vi "L5K Reader Action v2.vi"(8 "error in":errorcluster, 11 "L5K File Path":path) -> (0 "error out":errorcluster, 1 "Import Error":string, 3 "L5K Information":T1)   [LabVIEW 2011]
uses:
  L5K Internal Data.ctl
  L5K Tag.ctl
  L5K Data Types.ctl
  ST Enum.ctl
  Ethernet IP Custom Device Custom Device.lvlib
panel:
  out "concatenated string":string
  in  "Import Error - String":string="\n%s - Reason: this tag is a multidimensional array. VeriStand EtherNet/IP add-on only support 1D array tags."
  in  "Import Error - Array":string="\n%s - Reason: this tag is a multidimensional array. VeriStand EtherNet/IP add-on only support 1D array tags."
  in  "Import Error - Data Type":string="\n%s - Reason: the data type of this tag is not supported by the VeriStand EtherNet/IP add-on. Enter this tag manually with a generic datatype."
  in  "Import Error":string="VeriStand EtherNet/IP add-on did not import the following tags:\n"
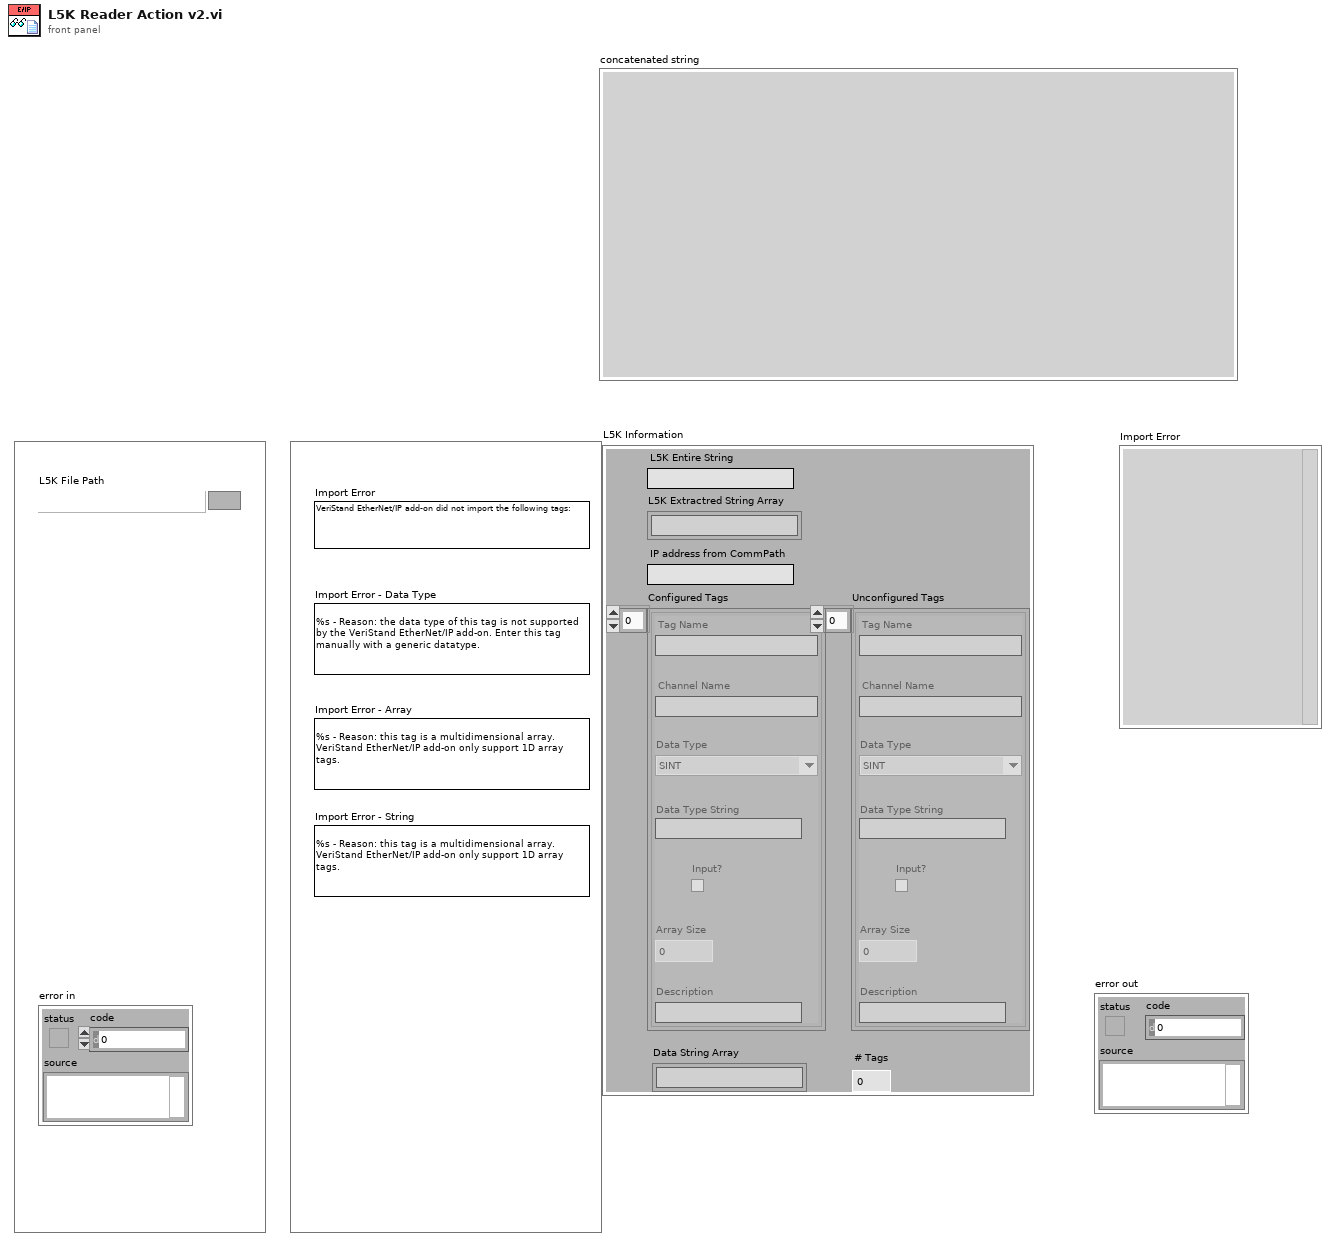
[diagram p1: front panel]
types:
  T1 = typedef "Ethernet IP Custom Device Custom Device.lvlib/L5K Internal Data.ctl" = cluster{"L5K Entire String":string, "L5K Extractred String Array":string[], "IP address from CommPath":string, "Configured Tags":T2[], "Data String Array":string[], "Unconfigured Tags":T2[], "# Tags":i32}
  T2 = typedef "Ethernet IP Custom Device Custom Device.lvlib/L5K Tag.ctl" = cluster{"Tag Name":string, "Data Type":T3, "Data Type String":string, "Array Size":i32, "Description":string, "Input?":bool, "Channel Name":string}
  T3 = typedef "Ethernet IP Custom Device Custom Device.lvlib/L5K Data Types.ctl" = enum16{"SINT", "INT", "DINT", "REAL", "BOOL"}
  T4 = typedef "Ethernet IP Custom Device Custom Device.lvlib/ST Enum.ctl" = enum16{"Init", "Extract Strings", "Extract Tags", "Exit"}
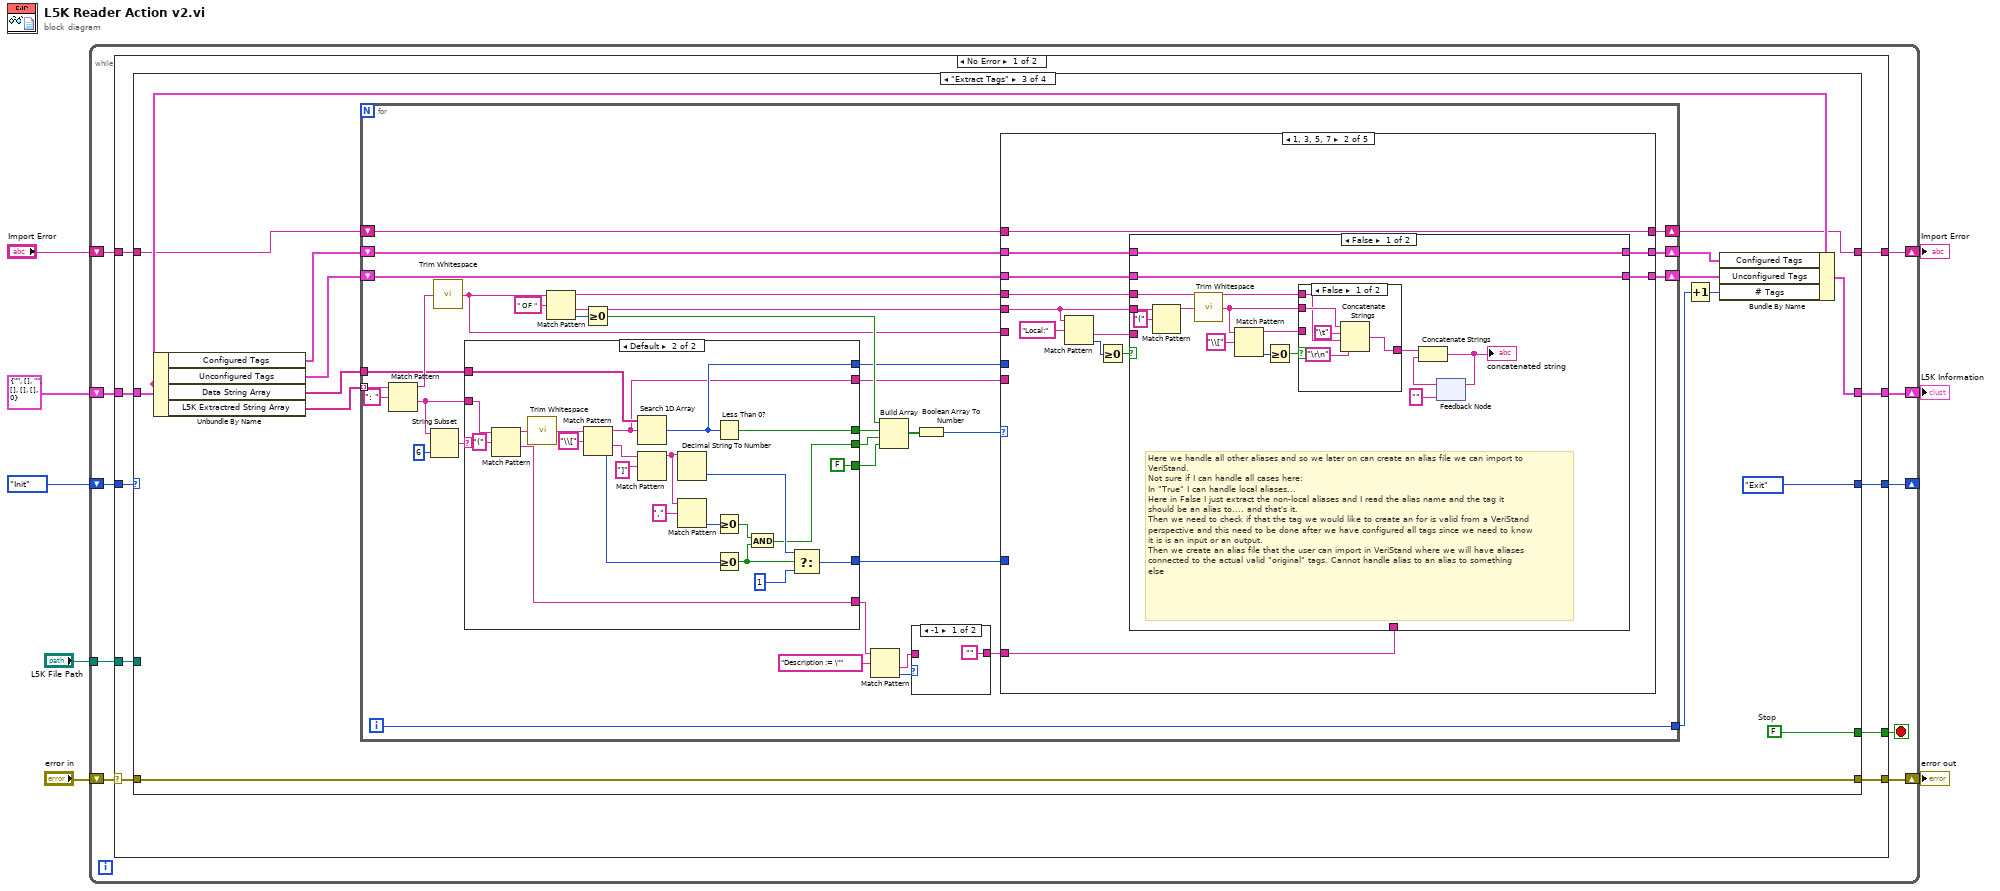
[diagram p0: block diagram]
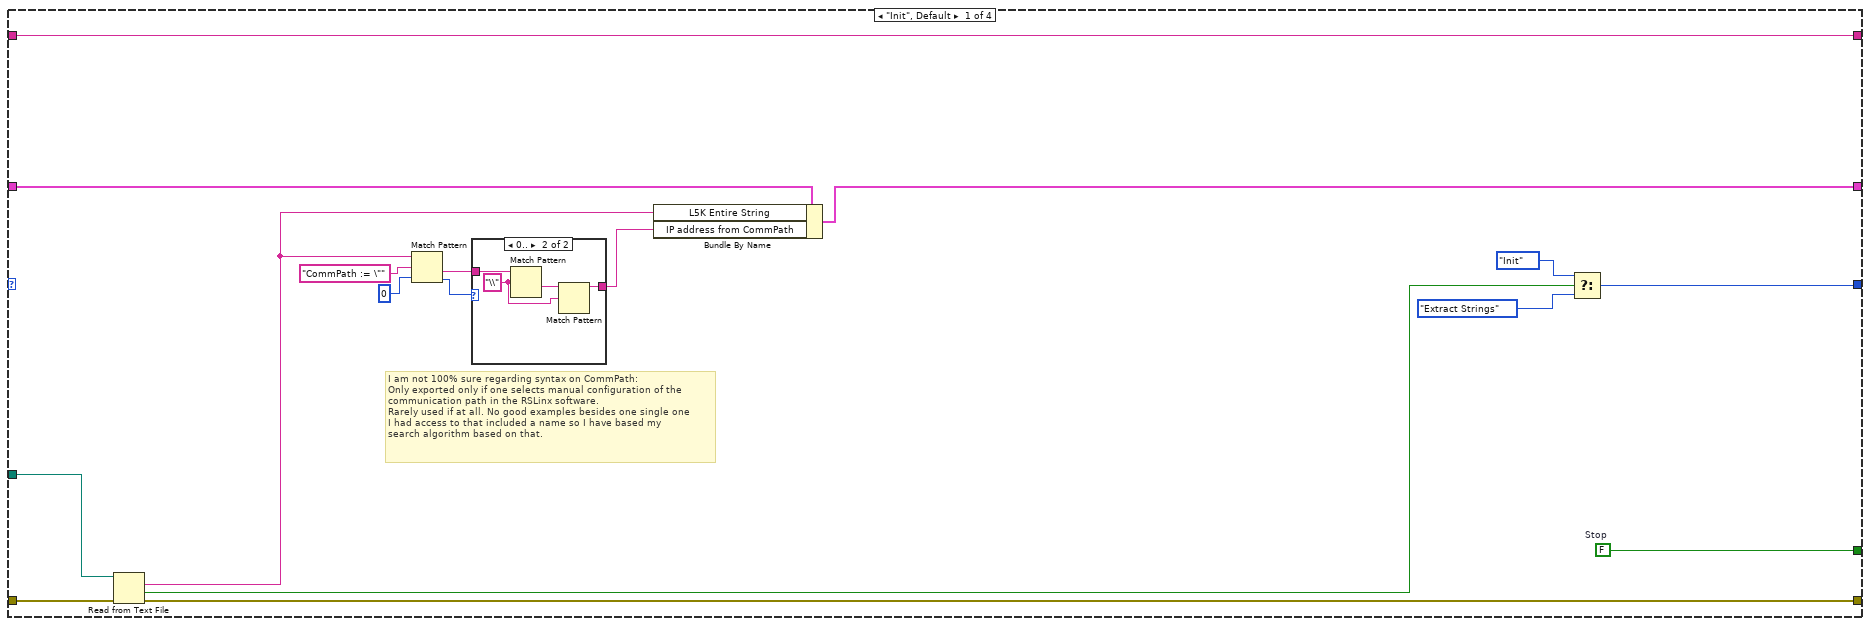
[diagram p2: hidden frame]
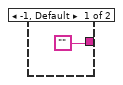
[diagram p3: hidden frame]
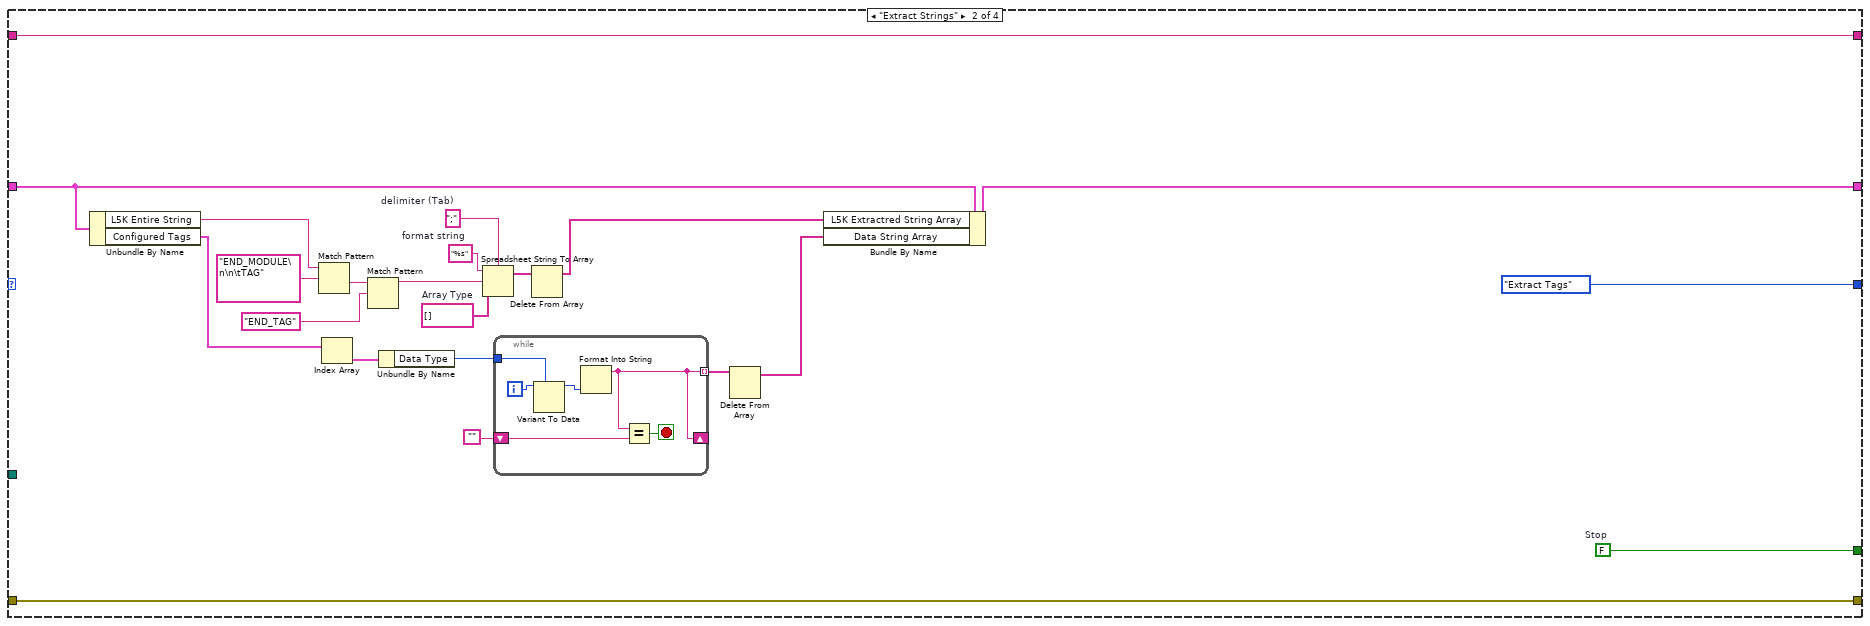
[diagram p4: hidden frame]
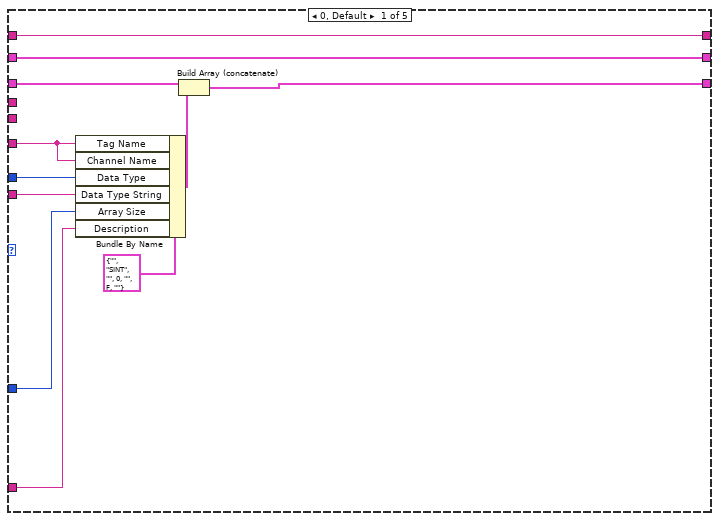
[diagram p5: hidden frame]
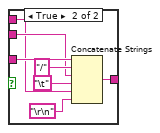
[diagram p6: hidden frame]
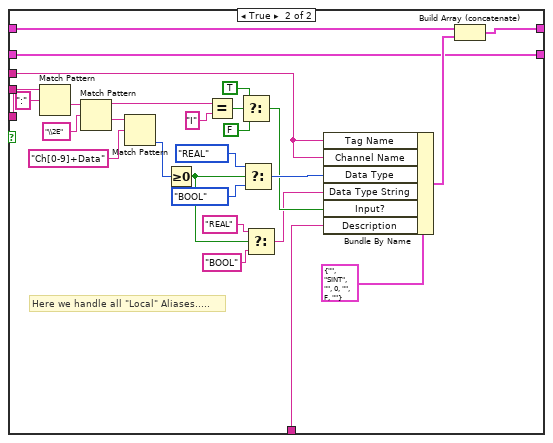
[diagram p7: hidden frame]
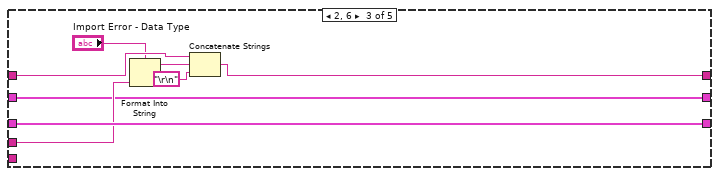
[diagram p8: hidden frame]
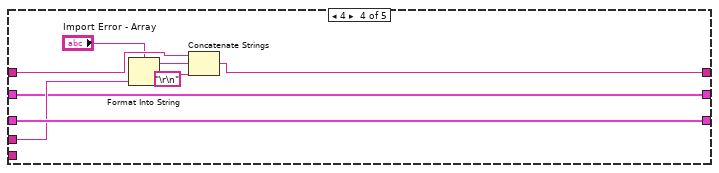
[diagram p9: hidden frame]
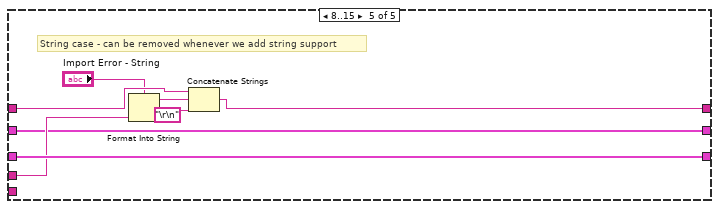
[diagram p10: hidden frame]
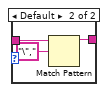
[diagram p11: hidden frame]
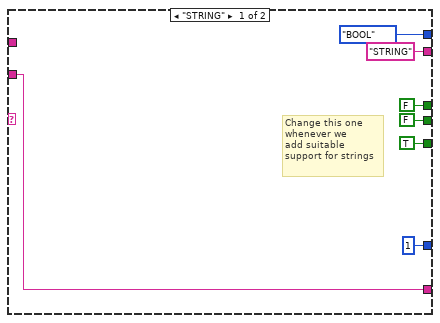
[diagram p12: hidden frame]
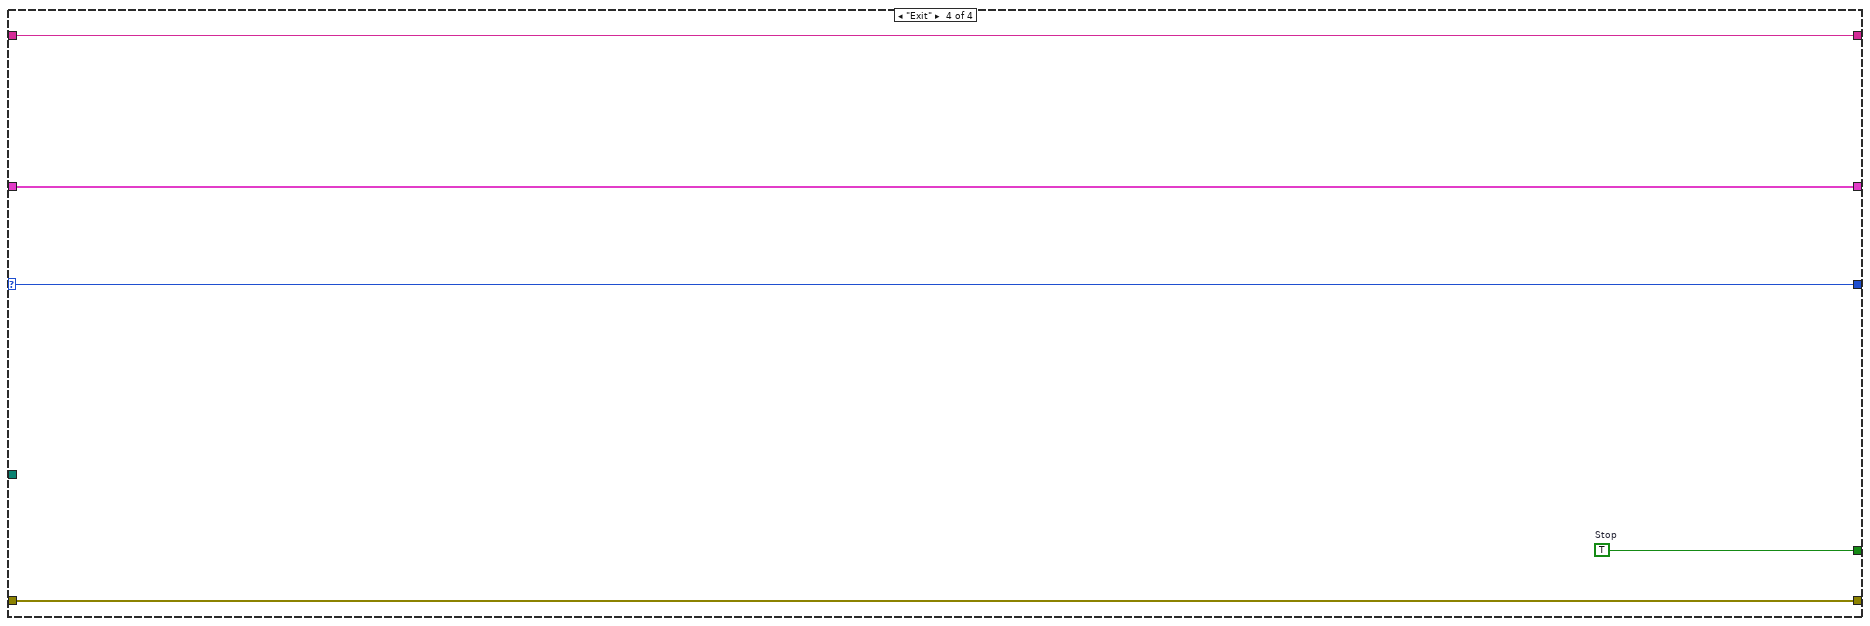
[diagram p13: hidden frame]
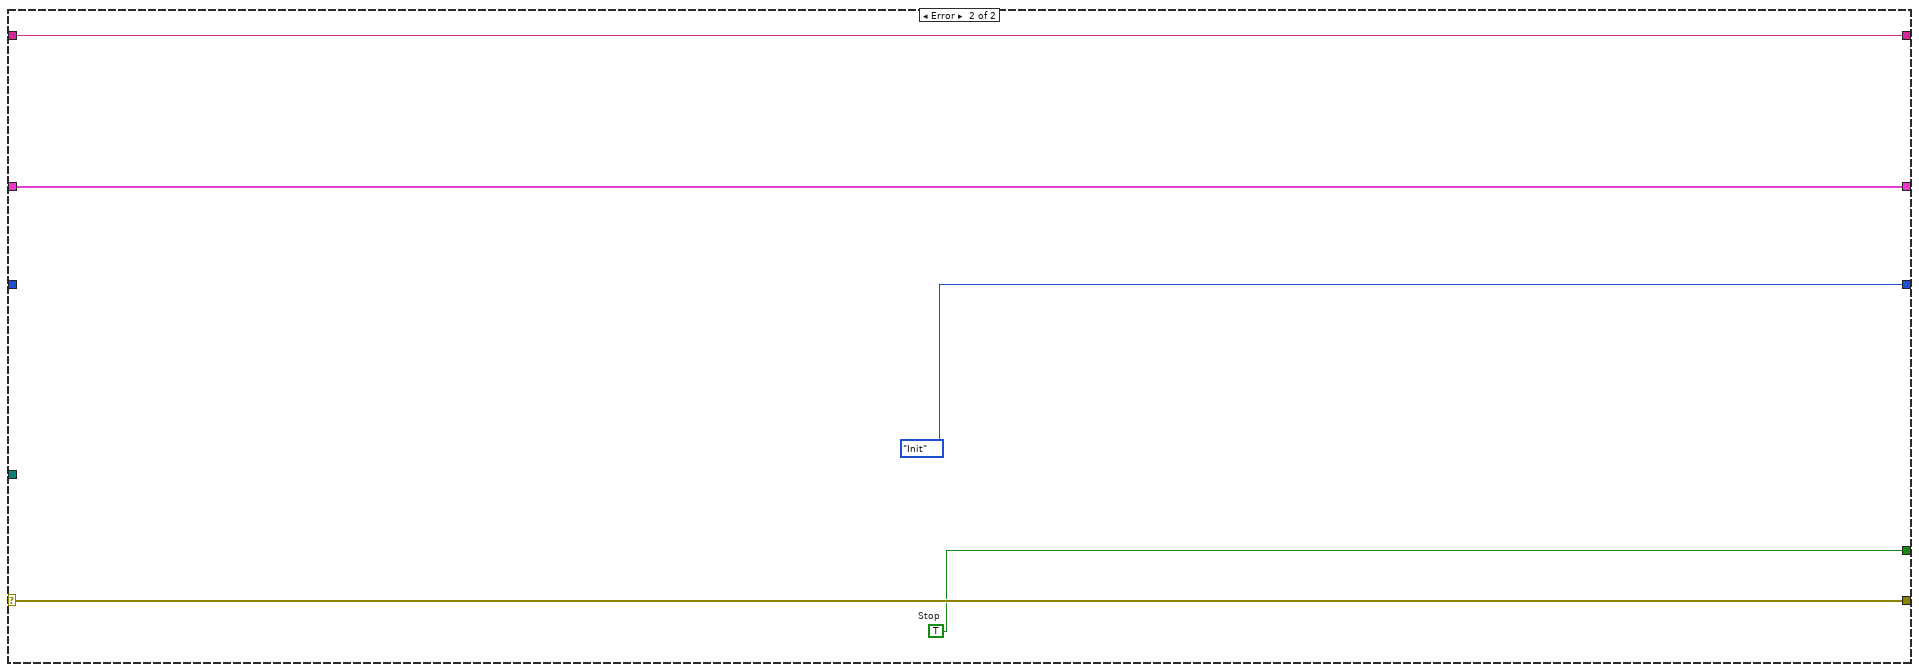
[diagram p14: hidden frame]
diagram:
  n1 = while {
    shift-right: [w16] -> _
    shift-left: ST_Enum."Init" ("Enum") -> [w18]
    shift-right: [w15] -> w5
    shift-left: "error in" -> [w12]
    shift-right: [w13] -> w1
    shift-left: T1 {"L5K Entire String"="", "L5K Extractred String Array"=[], "IP address from CommPath"="", "Configured Tags"=[], "Data String Array"=[], "Unconfigured Tags"=[], "# Tags"=0} ("L5K Information") -> [w14]
    shift-right: [w10] -> w3
    shift-left: "Import Error" -> [w11]
    tunnel: "L5K File Path" -> [w9]
    stop <- w17 stop-if-true
    n2 = case shown="No Error" w12 {
      selector: w12 -> [w22 w271]
      tunnel: w18 -> [w28 _]
      tunnel: [w27 w268] -> w17
      tunnel: [w26 ST_Enum."Init" ("Enum")] -> w16
      tunnel: [w25 w271] -> w15
      tunnel: w14 -> [w24 w270]
      tunnel: [w23 w270] -> w13
      tunnel: w11 -> [w21 w267]
      tunnel: [w20 w267] -> w10
      tunnel: w9 -> [w19 _]
      frame No Error {
        n3 = case shown="\"Extract Tags\"" w28 {
          selector: w28 -> [_ _ _ w265]
          tunnel: [w45 w59 w85 w266] -> w27
          tunnel: [w44 ST_Enum."Extract Tags" ("Enum") ST_Enum."Exit" ("Enum") w265] -> w26
          tunnel: w22 -> [w43 w60 w86 w264]
          tunnel: [w42 w60 w86 w264] -> w25
          tunnel: w24 -> [w41 w63 w90 w263]
          tunnel: [w40 w61 w88 w263] -> w23
          tunnel: w21 -> [w39 w51 w84 w262]
          tunnel: [w39 w51 w83 w262] -> w20
          tunnel: w19 -> [w35 _ _ _]
          frame "Init", Default {
            w45 = FALSE  # Stop
            # "I am not 100% sure regarding syntax on CommPath:\nOnly exported only if one selects manual configuration of the \ncommunication path in the RSLinx software.\nRarely used if at all. No good examples besides one single one\nI had access to that included a name so I have based my\nsearch algorithm based on that."
            n4 = Read from Text File(file (use dialog)=w35, error in=w43) -> (text=w30:string, cancelled=w38:bool, error out=w42:errorcluster)  [unwired: 2 in, 1 out]
            n5 = Match Pattern(string=w30, regular expression="CommPath := \"", offset (0)=0) -> (after substring=w33:string, offset past match=w32:i32)  [unwired: 2 out]
            n6 = case shown="0.." w32 {
              tunnel: w33 -> [_ w50]
              tunnel: ["" w47] -> w29
              frame -1, Default {
              }
              frame 0.. {
                w48 = "\\" ("regular expression")
                n7 = Match Pattern(string=w50, regular expression=w48) -> (after substring=w49:string)  [unwired: 1 in, 3 out]
                n8 = Match Pattern(string=w49, regular expression=w48) -> (before substring=w47:string)  [unwired: 1 in, 3 out]
              }
            }
            n9 = Bundle By Name(cluster=w41, "L5K Entire String"=w30, "IP address from CommPath"=w29) -> (w40:T1)
            n10 = Select(t=ST_Enum."Init" ("Enum"), s=w38, f=ST_Enum."Extract Strings" ("Enum")) -> (s? t:f=w44:T4)
          }
          frame "Extract Strings" {
            w59 = FALSE  # Stop
            w71 = string[] []  # Array Type
            w70 = ";"  # delimiter (Tab)
            w69 = "%s"  # format string
            n11 = Unbundle By Name(w63) -> ("L5K Entire String"=w64:string, "Configured Tags"=w57:T2[])
            n12 = Match Pattern(string=w64, regular expression="END_MODULE\n\n\tTAG") -> (after substring=w66:string)  [unwired: 1 in, 3 out]
            n13 = Index Array(array=w57) -> (element=w56:T2)  [unwired: 1 in]
            n14 = Match Pattern(string=w66, regular expression="END_TAG") -> (before substring=w68:string)  [unwired: 1 in, 3 out]
            n15 = Unbundle By Name(w56) -> ("Data Type"=w54:T3)
            n16 = Spreadsheet String To Array(delimiter (Tab)=w70, format string=w69, spreadsheet string=w68, array type (2D Dbl)=w71) -> (array=w72:string[])
            n17 = while {
              shift-right: [w73] -> _
              shift-left: "" -> [w77]
              tunnel: w54 -> [w76]
              tunnel: [w73] -> w53 mode=indexing
              i -> [w75]
              stop <- w78 stop-if-true
              n18 = Variant To Data(type=w76, Variant=w75) -> (data=w74:T3)  [unwired: 1 in, 1 out]
              n19 = Format Into String(w74) -> (resulting string=w73:string)  [unwired: 3 in, 1 out]
              n20 = Equal?(x=w73, y=w77) -> (x = y?=w78:bool)
            }
            n21 = Delete From Array(array=w72) -> (array with subset deleted=w62:string[])  [unwired: 2 in, 1 out]
            n22 = Delete From Array(array=w53) -> (array with subset deleted=w52:string[])  [unwired: 2 in, 1 out]
            n23 = Bundle By Name(cluster=w63, "L5K Extractred String Array"=w62, "Data String Array"=w52) -> (w61:T1)
          }
          frame "Extract Tags" {
            w85 = FALSE  # Stop
            n24 = Unbundle By Name(w90) -> ("Configured Tags"=w82:T2[], "Unconfigured Tags"=w91:T2[], "Data String Array"=w92:string[], "L5K Extractred String Array"=w93:string[])
            n25 = for {
              tunnel: w93 -> [w123] mode=indexing
              tunnel: w92 -> [w120]
              shift-right: [w103] -> w89
              shift-left: w91 -> [w104]
              shift-right: [w101] -> w83
              shift-left: w84 -> [w100]
              shift-right: [w96] -> w81
              shift-left: w82 -> [w97]
              tunnel: [w95] -> w79
              i -> [w95]
              n26 = Match Pattern(string=w123, regular expression=": ") -> (before substring=w125:string, after substring=w121:string)  [unwired: 1 in, 2 out]
              n27 = String Subset(string=w121, length (rest)=6 ("length (rest)")) -> (substring=w122:string)  [unwired: 1 in]
              n28 = call <vilib>:"Trim Whitespace.vi"("string"=w125) -> ("trimmed string"=w108:string)  [unwired: 1 in]
              n29 = case shown="Default" w122 {
                tunnel: w121 -> [w238 w248]
                tunnel: w120 -> [_ w246]
                tunnel: [w238 w245] -> w114
                tunnel: [FALSE w244] -> w112
                tunnel: [FALSE w243] -> w111
                tunnel: [L5K_Data_Types."BOOL" ("Data Type") w242] -> w107
                tunnel: [1 ("t") w241] -> w106
                tunnel: ["STRING" ("trimmed string") w240] -> w99
                tunnel: [TRUE FALSE] -> w94
                frame "STRING" {
                  # "Change this one\nwhenever we\nadd suitable\nsupport for strings"
                }
                frame Default {
                  n30 = Match Pattern(string=w248, regular expression="(") -> (before substring=w250:string, after substring=w245:string)  [unwired: 1 in, 2 out]
                  n31 = call <vilib>:"Trim Whitespace.vi"("string"=w250) -> ("trimmed string"=w251:string)  [unwired: 1 in]
                  n32 = Match Pattern(string=w251, regular expression="\\[") -> (before substring=w240:string, after substring=w253:string, offset past match=w257:i32)  [unwired: 1 in, 1 out]
                  n33 = Search 1D Array(1D array=w246, element=w240) -> (index of element=w242:i32)  [unwired: 1 in]
                  n34 = Match Pattern(string=w253, regular expression="]") -> (before substring=w256:string)  [unwired: 1 in, 3 out]
                  n35 = Decimal String To Number(string=w256) -> (number=w249:i32)  [unwired: 2 in, 1 out]
                  n36 = Match Pattern(string=w256, regular expression=",") -> (offset past match=w259:i32)  [unwired: 1 in, 3 out]
                  n37 = Less Than 0?(x=w242) -> (x < 0?=w243:bool)
                  n38 = Greater Or Equal To 0?(x=w259) -> (x >= 0?=w260:bool)
                  n39 = Greater Or Equal To 0?(x=w257) -> (x >= 0?=w261:bool)
                  n40 = And(x=w260, y=w261) -> (x .and. y?=w244:bool)
                  n41 = Select(t=w249, s=w261, f=1 ("t")) -> (s? t:f=w241:i32)
                }
              }
              n42 = Match Pattern(string=w108, regular expression=" OF ") -> (before substring=w102:string, after substring=w98:string, offset past match=w118:i32)  [unwired: 1 in, 1 out]
              n43 = Greater Or Equal To 0?(x=w118) -> (x >= 0?=w110:bool)
              n44 = Match Pattern(string=w114, regular expression="Description := \"") -> (after substring=w115:string, offset past match=w116:i32)  [unwired: 1 in, 2 out]
              n45 = Build Array(w110, w111, w112, w94) -> (w113:bool[])
              n46 = case shown="-1" w116 {
                tunnel: ["" w230] -> w105
                tunnel: w115 -> [_ w229]
                frame -1 {
                }
                frame Default {
                  n47 = Match Pattern(string=w229, regular expression="\",") -> (before substring=w230:string)  [unwired: 1 in, 3 out]
                }
              }
              n48 = Boolean Array To Number(Boolean array=w113) -> (number=w109:u32)
              n49 = case shown="1, 3, 5, 7" w109 {
                tunnel: w108 -> [w127 _ _ _ _]
                tunnel: w107 -> [w136 _ _ _ _]
                tunnel: w106 -> [w130 _ _ _ _]
                tunnel: w105 -> [w135 w148 _ _ _]
                tunnel: w104 -> [w134 w139 w211 w219 w227]
                tunnel: [w132 w138 w211 w219 w227] -> w103
                tunnel: w102 -> [_ w147 w207 w215 w223]
                tunnel: [w131 w149 w210 w218 w226] -> w101
                tunnel: w100 -> [w131 w149 w208 w216 w224]
                tunnel: w99 -> [w129 _ _ _ _]
                tunnel: w98 -> [_ w142 _ _ _]
                tunnel: w97 -> [w128 w140 w204 w212 w220]
                tunnel: [w128 w141 w204 w212 w220] -> w96
                frame 0, Default {
                  n50 = Bundle By Name(cluster=T2 {"Tag Name"="", "Data Type"=enum."SINT", "Data Type String"="", "Array Size"=0, "Description"="", "Input?"=FALSE, "Channel Name"=""} ("Tag"), "Tag Name"=w127, "Channel Name"=w127, "Data Type"=w136, "Data Type String"=w129, "Array Size"=w130, "Description"=w135) -> (w133:T2)
                  n51 = Build Array (concatenate)(w134, w133) -> (w132:T2[])
                }
                frame 1, 3, 5, 7 {
                  n52 = Match Pattern(string=w142, regular expression="Local:") -> (after substring=w145:string, offset past match=w144:i32)  [unwired: 1 in, 2 out]
                  n53 = Greater Or Equal To 0?(x=w144) -> (x >= 0?=w143:bool)
                  n54 = case shown="False" w143 {
                    tunnel: w148 -> [_ w187]
                    tunnel: w147 -> [w153 w182]
                    tunnel: w145 -> [_ w181]
                    tunnel: w142 -> [w163 _]
                    tunnel: [w161 w179] -> w141
                    tunnel: w140 -> [w161 w178]
                    tunnel: w139 -> [w160 w177]
                    tunnel: [w160 w177] -> w138
                    frame False {
                      # "Here we handle all other aliases and so we later on can create an alias file we can import to VeriStand.\nNot sure if I can handle all cases here:\nIn \"True\" I can handle local aliases...\nHere in False I just extract the non-local aliases and I read the alias name and the tag it should be an alias to.... and that's it. \nThen we need to check if that the tag we would like to create an for is valid from a VeriStand perspective and this need to be done after we have configured all tags since we need to know it is is an input or an output.\nThen we create an alias file that the user can import in VeriStand where we will have aliases connected to the actual valid \"original\" tags. Cannot handle alias to an alias to something else"
                      n55 = Match Pattern(string=w163, regular expression="(") -> (before substring=w162:string)  [unwired: 1 in, 3 out]
                      n56 = call <vilib>:"Trim Whitespace.vi"("string"=w162) -> ("trimmed string"=w154:string)  [unwired: 1 in]
                      n57 = Match Pattern(string=w154, regular expression="\\[") -> (before substring=w155:string, offset past match=w157:i32)  [unwired: 1 in, 2 out]
                      n58 = Greater Or Equal To 0?(x=w157) -> (x >= 0?=w156:bool)
                      n59 = case shown="False" w156 {
                        tunnel: w155 -> [_ w176]
                        tunnel: w154 -> [w169 w174]
                        tunnel: w153 -> [w167 w172]
                        tunnel: [w165 w170] -> w152
                        frame False {
                          n60 = Concatenate Strings(w169, "\t", w167, "\r\n") -> (w165:string)
                        }
                        frame True {
                          n61 = Concatenate Strings(w176, "/" ("string"), w174, "\t", w172, "\r\n") -> (w170:string)
                        }
                      }
                      n62 = feedback #1("") -> (w150:string)
                      n63 = Concatenate Strings(w152, w150) -> (w151:string)
                      "concatenated string" <- w151
                      n64 = feedback-in #1(w151) -> ()
                    }
                    frame True {
                      # "Here we handle all \"Local\" Aliases....."
                      n65 = Match Pattern(string=w181, regular expression=":") -> (after substring=w199:string)  [unwired: 1 in, 3 out]
                      n66 = Match Pattern(string=w199, regular expression="\\2E") -> (before substring=w191:string, after substring=w198:string)  [unwired: 1 in, 2 out]
                      n67 = Match Pattern(string=w198, regular expression="Ch[0-9]+Data") -> (offset past match=w196:i32)  [unwired: 1 in, 3 out]
                      n68 = Greater Or Equal To 0?(x=w196) -> (x >= 0?=w186:bool)
                      n69 = Equal?(x=w191, y="I") -> (x = y?=w202:bool)
                      n70 = Select(t=TRUE, s=w202, f=FALSE) -> (s? t:f=w188:bool)
                      n71 = Select(t=L5K_Data_Types."REAL" ("Data Type"), s=w186, f=L5K_Data_Types."BOOL" ("Data Type")) -> (s? t:f=w195:T3)
                      n72 = Select(t="REAL", s=w186, f="BOOL") -> (s? t:f=w183:string)
                      n73 = Bundle By Name(cluster=T2 {"Tag Name"="", "Data Type"=enum."SINT", "Data Type String"="", "Array Size"=0, "Description"="", "Input?"=FALSE, "Channel Name"=""} ("Tag"), "Tag Name"=w182, "Channel Name"=w182, "Data Type"=w195, "Data Type String"=w183, "Input?"=w188, "Description"=w187) -> (w180:T2)
                      n74 = Build Array (concatenate)(w178, w180) -> (w179:T2[])
                    }
                  }
                }
                frame 2, 6 {
                  n75 = Format Into String(format string="Import Error - Data Type", w207) -> (resulting string=w209:string)  [unwired: 2 in, 1 out]
                  n76 = Concatenate Strings(w208, w209, "\r\n") -> (w210:string)
                }
                frame 4 {
                  n77 = Format Into String(format string="Import Error - Array", w215) -> (resulting string=w217:string)  [unwired: 2 in, 1 out]
                  n78 = Concatenate Strings(w216, w217, "\r\n") -> (w218:string)
                }
                frame 8..15 {
                  # "String case - can be removed whenever we add string support"
                  n79 = Format Into String(format string="Import Error - String", w223) -> (resulting string=w225:string)  [unwired: 2 in, 1 out]
                  n80 = Concatenate Strings(w224, w225, "\r\n") -> (w226:string)
                }
              }
            }
            n81 = Increment(x=w79) -> (x+1=w80:i32)
            n82 = Bundle By Name(cluster=w90, "Configured Tags"=w81, "Unconfigured Tags"=w89, "# Tags"=w80) -> (w88:T1)
          }
          frame "Exit" {
            w266 = TRUE  # Stop
          }
        }
      }
      frame Error {
        w268 = TRUE  # Stop
      }
    }
  }
  "error out" <- w5
  "Import Error" <- w3
  "L5K Information" <- w1
